vi "Solve1.vi"(8 "Error In":errorcluster, 11 "object in":refnum<class "2021_15.lvclass">) -> (0 "Error Out":errorcluster, 2 "Result":u64, 3 "object out":refnum<class "2021_15.lvclass">)   [LabVIEW 2020, in "2021_15.lvclass"]
uses:
  2021_15.lvclass
  2021_15.lvclass/2021_15.ctl
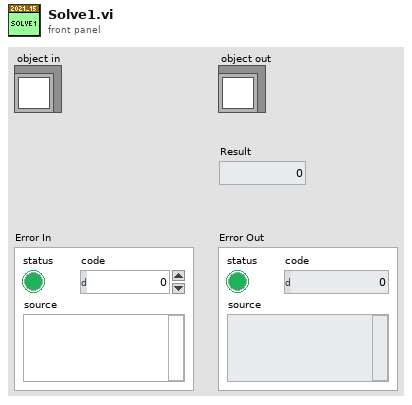
[diagram p1: front panel]
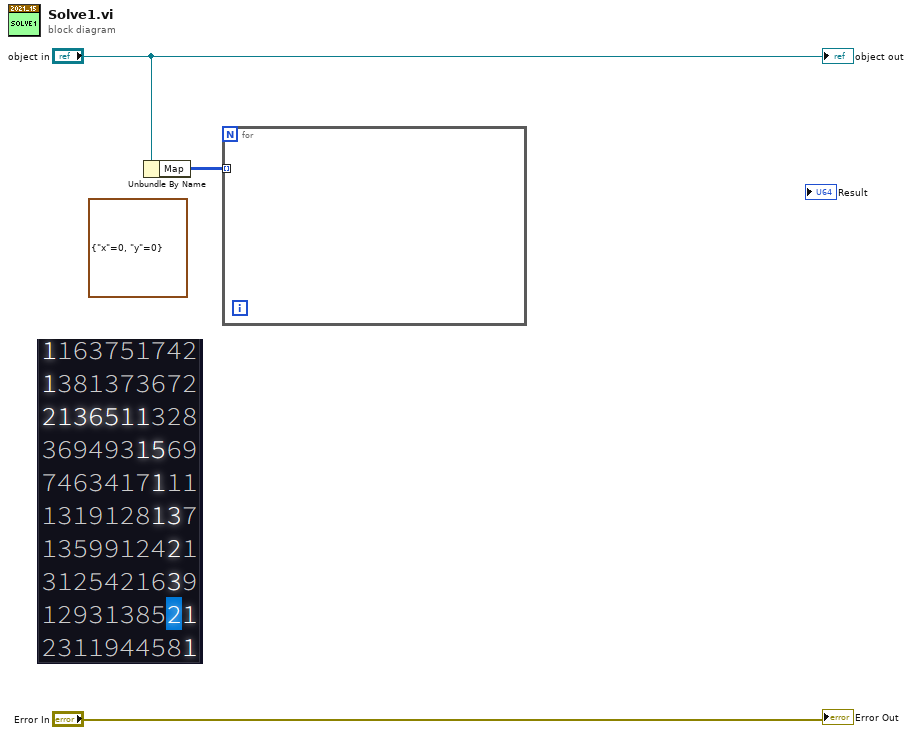
[diagram p0: block diagram]
diagram:
  (unwired) cluster{"x":i32, "y":i32} {"x"=0, "y"=0}
  n1 = Unbundle By Name("object in") -> ("Map"=w1:u8[][])
  n2 = for {
    tunnel: w1 -> [_] mode=indexing
  }
  "Error Out" <- "Error In"
  "object out" <- "object in"
